vi "Run.vi"(6 "Type y_pred":T2(ring), 7 "Type y_true":T2(ring), 8 "error in (no error)":errorcluster caption="entrée d'erreur (pas d'erreur)", 9 "y_pred":string[][](array[string]), 10 "y_true":string[][](array[string]), 11 "Multilabel_Confusion_Matrix.lvclass":refnum<class "Multilabel_Confusion_Matrix.lvclass">) -> (0 "error out":errorcluster caption="sortie d'erreur", 2 "Data":T1, 3 "Multilabel_Confusion_Matrix.lvclass":refnum<class "Multilabel_Confusion_Matrix.lvclass">)   [LabVIEW 2020, in "Multilabel_Confusion_Matrix.lvclass"]
doc: "Returns :\n\n- multi_confusion : array, shape (n_outputs, 2, 2)\nA 2x2 confusion matrix corresponding to each output in the input. When calculating class-wise multi_confusion (default), then n_outputs = n_labels; when calculating sample-wise multi_confusion (samplewise=True), n_outputs = n_samples. If labels is defined, the results will be returned in the order specified in labels, otherwise the results will be returned in sorted order by default."
uses:
  Multilabel_Confusion_Matrix.lvclass
  Multilabel_Confusion_Matrix.lvclass/Multilabel_Confusion_Matrix.ctl
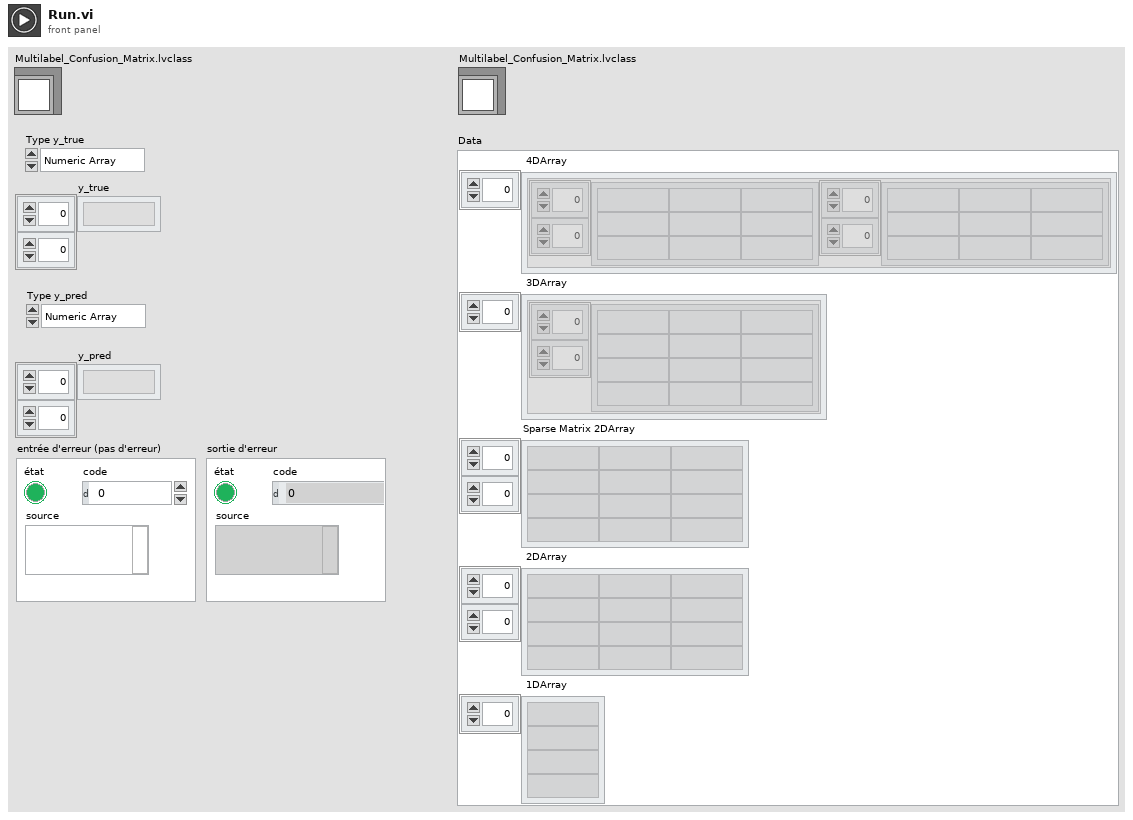
[diagram p1: front panel]
types:
  T1 = cluster{" 4DArray":cluster{"1":string[][], "2":string[][]}[], " 3DArray":cluster{"Tableau":string[][]}[], "Sparse Matrix 2DArray":string[][], " 2DArray":string[][], " 1DArray":string[]}
  T2 = enum16{"Numeric Array", "String Array", "Sparse"}
  T3 = cluster{"dtype_labels":string, "labels":string[]}
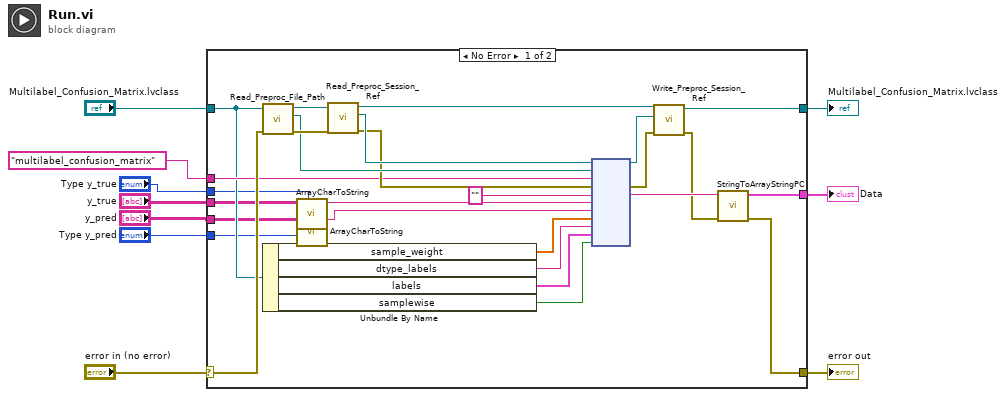
[diagram p0: block diagram]
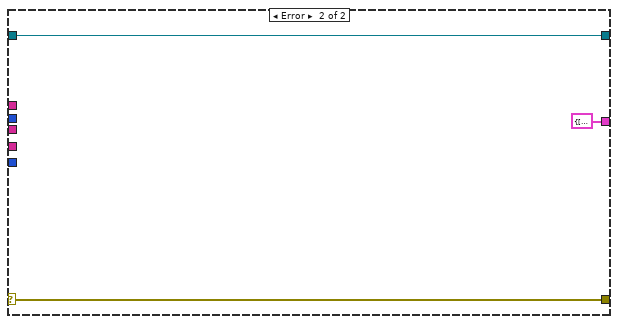
[diagram p2: hidden frame]
diagram:
  n1 = case shown="No Error" "error in (no error)" {
    selector: "error in (no error)" -> [w28 w40]
    tunnel: [w12 w40] -> w9
    tunnel: [w15 w39] -> w7
    tunnel: "Multilabel_Confusion_Matrix.lvclass" -> [w26 w39]
    tunnel: "multilabel_confusion_matrix" -> [w27 _]
    tunnel: "y_true" -> [w21 _]
    tunnel: "y_pred" -> [w19 _]
    tunnel: "Type y_true" -> [w20 _]
    tunnel: "Type y_pred" -> [w18 _]
    tunnel: [w11 T1 {" 4DArray"=[], " 3DArray"=[], "Sparse Matrix 2DArray"=[], " 2DArray"=[], " 1DArray"=[]} ("Data")] -> w1
    frame No Error {
      n2 = call-dynamic "Read_Preproc_File_Path.vi"("error in (no error)"=w28, "Python in"=w26) -> ("error out"=w36:errorcluster, "File_Path"=w35:path, "Python out"=w37:refnum<class "Multilabel_Confusion_Matrix.lvclass">)  [unwired: 7 in]
      n3 = Unbundle By Name(w26) -> ("sample_weight"=w25:dbl[], "dtype_labels"=w24:string, "labels"=w23:T3, "samplewise"=w22:bool)
      n4 = call "ArrayCharToString.vi"("Type"=w20, "TAB"=w21) -> ("Instruction"=w17:string)  [unwired: 9 in]
      n5 = call "ArrayCharToString.vi"("Type"=w18, "TAB"=w19) -> ("Instruction"=w16:string)  [unwired: 9 in]
      n6 = call-dynamic "Read_Preproc_Session_Ref.vi"("error in (no error)"=w36, "Python in"=w37) -> ("error out"=w33:errorcluster, "Session_ref"=w34:refnum<k35>, "Python out"=w32:refnum<class "Multilabel_Confusion_Matrix.lvclass">)  [unwired: 7 in]
      n7 = node(w34, w35, w27, w33, "", w17, w16, w25, w24, w23, w22) -> (w30:refnum<k35>, w31:errorcluster, w14:string)  [unwired: 6 in, 2 out]
      n8 = call-dynamic "Write_Preproc_Session_Ref.vi"("error in (no error)"=w31, "Session_ref"=w30, "Python in"=w32) -> ("error out"=w13:errorcluster, "Python out"=w15:refnum<class "Multilabel_Confusion_Matrix.lvclass">)  [unwired: 7 in]
      n9 = call "StringToArrayStringPC.vi"("sortie d'erreur"=w13, "Return value"=w14) -> ("sortie d'erreur"=w12:errorcluster, "Data"=w11:T1)  [unwired: 8 in]
    }
    frame Error {
    }
  }
  "error out" <- w9
  "Multilabel_Confusion_Matrix.lvclass" <- w7
  "Data" <- w1
